vi "Clipper.vi"(8 "error in (no error)":errorcluster) -> (0 "error out":errorcluster)   [LabVIEW 2018, in "MainVIs.lvlib"]
doc: "This template is for the Queued Message Handler design pattern.\n\nThe Event Handling Loop generates messages based on user interface actions.\n\nThe Message Handling Loop processes messages generated by the Event Handling Loop, or by other messages. The messages are string values, so new messages can be added easily to the Message Cases case structure in the Message Handling Loop. Each message cluster can also provide an optional value for Message Data, which is a variant that can be converted to whatever message-specific data is required."
uses:
  MainVIs.lvlib
  <vilib>/Utility/miscctls.llb/LVCursorListTypeDef.ctl
  Analysis Support/Controls/UI Data-Clipper.ctl
  Collection Support/Message Queue/Enqueue Message (Single).vi
  Collection Support/Message Queue/Enqueue Message (Array).vi
  <vilib>/Utility/error.llb/Error Cluster From Error Code.vi
  <vilib>/ErrorRing/Error Ring.xnode
  Collection Support/Message Queue/Message Queue.lvlib
  Collection Support/User Event - Stop/User Event - Stop.lvlib
  CollectionSupport.lvlib
  AnalysisSupport.lvlib
panel:
  in  "Stop Everything?":bool
  out "Right":dbl
  out "Left":dbl
  out "Flow":dynamicdata(graph)
  out "Pressure":dynamicdata(graph)
  out "Audio":dynamicdata(graph)
  out "File Name Display":string
  in  "Remove":bool
  in  "Set Cursors":bool
  in  "Edit File":bool
  out "Message":string
  in  "Save":bool
  in  "Open":bool
  in  "Exit":bool
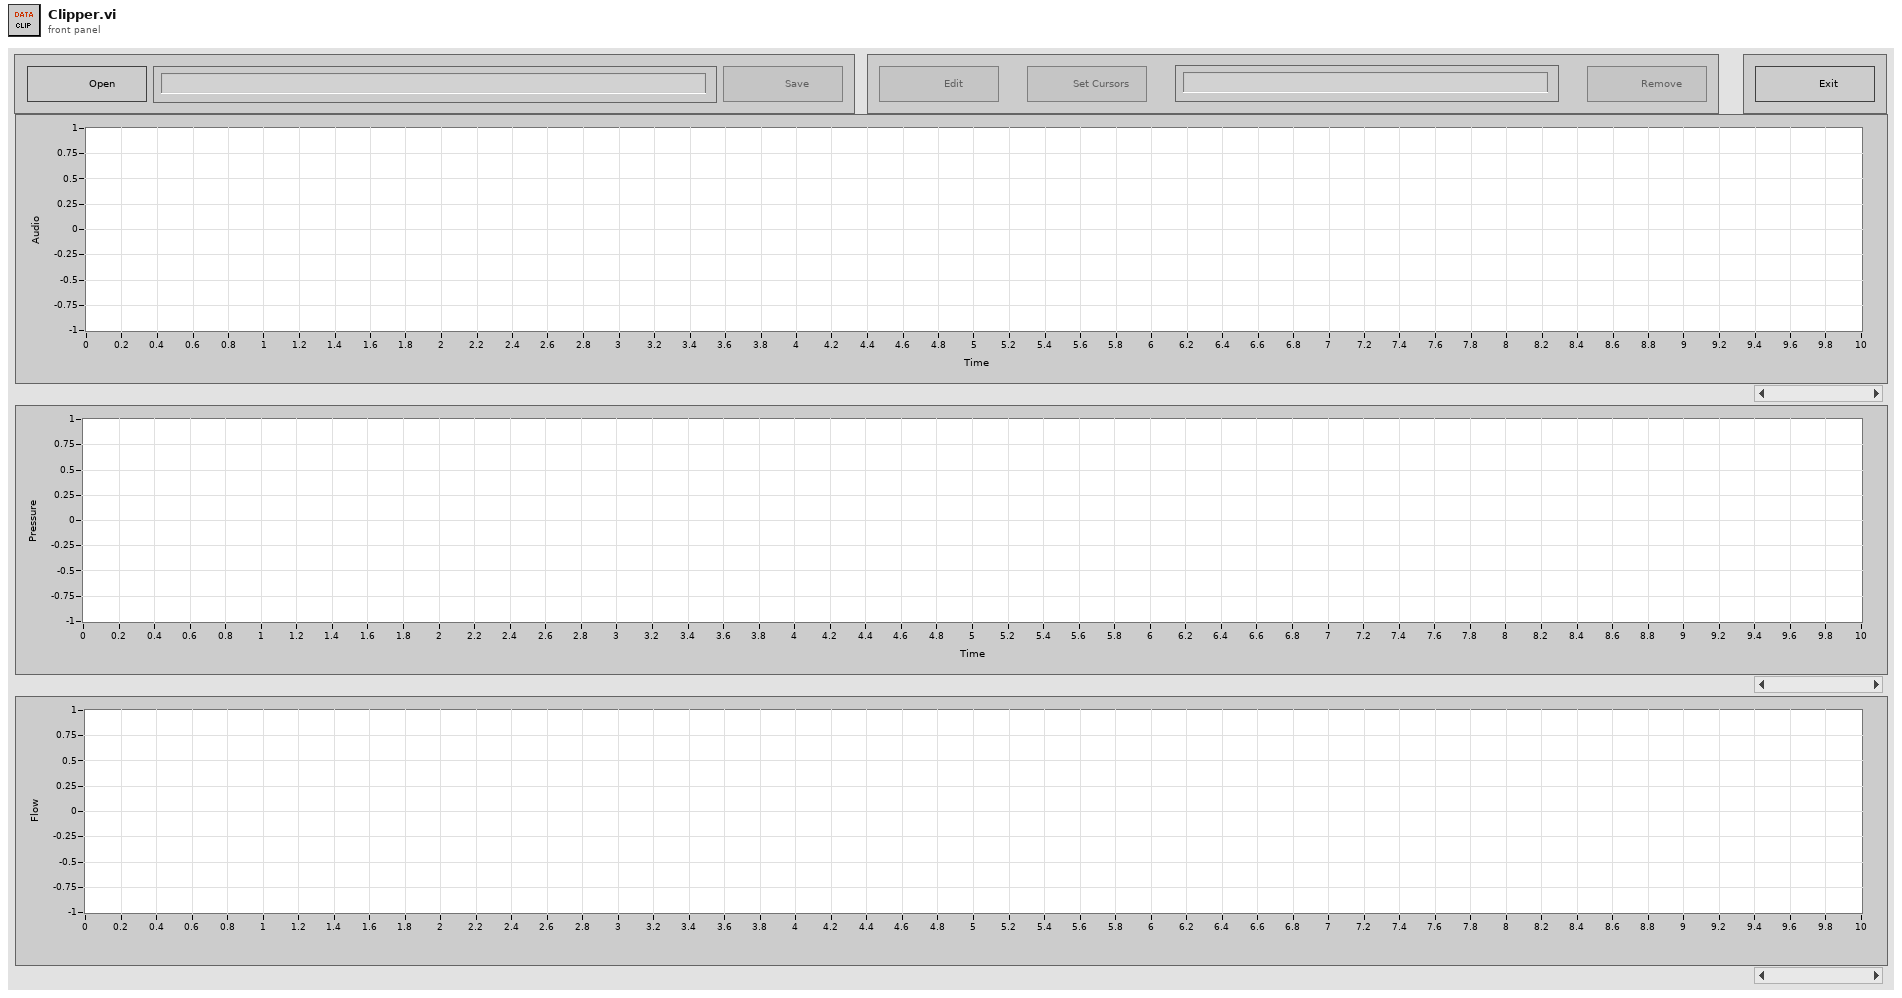
[diagram p1: front panel]
types:
  T1 = typedef "AnalysisSupport.lvlib/UI Data-Clipper.ctl" = cluster{"File Loaded?":bool, "Message":string, "Open Ref":refnum<vi>, "Save Ref":refnum<vi>, "Message Ref":refnum<vi>, "Exit Button Ref":refnum<vi>, "Remove Ref":refnum<vi>, "Set Cursors Ref":refnum<vi>, "Edit File Ref":refnum<vi>, "Audio Ref":refnum<vi>, "Pressure Ref":refnum<vi>, "Flow Ref":refnum<vi>, "Audio":dynamicdata, "Pressure":dynamicdata, "Flow":dynamicdata, "Left Cursor Position":dbl, "Right Cursor Position":dbl, "Cursors Locked?":bool, "File Name Display":string}
  T2 = typedef "LVCursorListTypeDef.ctl" = cluster{"Name":string, "Color":u32, "Style":u8, "Point Style":u8, "Name Visible":bool, "Allow Drag":bool, "Cursor Mode":u32, "Plot":i32, "Index":i32, "Position":cluster{"X":dbl, "Y":dbl}, "X Scale":u32, "Y Scale":u32, "Watch Plots":i32[], "Watch All Plots":bool, "Plot Area":i32, "Label Offset":cluster{"X":dbl, "Y":dbl}}[]
  T3 = typedef "CollectionSupport.lvlib/Message Queue.lvlib/All Message Queues.ctl" = cluster{"UI":refnum<queue>}
  T4 = cluster{"Cursor Constants[0]":cluster{"Name":string, "Color":u32, "Style":u8, "Point Style":u8, "Name Visible":bool, "Allow Drag":bool, "Cursor Mode":u32, "Plot":i32, "Index":i32, "Position":cluster{"X":dbl, "Y":dbl}, "X Scale":u32, "Y Scale":u32, "Watch Plots":i32[], "Watch All Plots":bool, "Plot Area":i32, "Label Offset":cluster{"X":dbl, "Y":dbl}}, "Cursor Constants[1]":cluster{"Name":string, "Color":u32, "Style":u8, "Point Style":u8, "Name Visible":bool, "Allow Drag":bool, "Cursor Mode":u32, "Plot":i32, "Index":i32, "Position":cluster{"X":dbl, "Y":dbl}, "X Scale":u32, "Y Scale":u32, "Watch Plots":i32[], "Watch All Plots":bool, "Plot Area":i32, "Label Offset":cluster{"X":dbl, "Y":dbl}}, "Cursor Constants[2]":cluster{"Name":string, "Color":u32, "Style":u8, "Point Style":u8, "Name Visible":bool, "Allow Drag":bool, "Cursor Mode":u32, "Plot":i32, "Index":i32, "Position":cluster{"X":dbl, "Y":dbl}, "X Scale":u32, "Y Scale":u32, "Watch Plots":i32[], "Watch All Plots":bool, "Plot Area":i32, "Label Offset":cluster{"X":dbl, "Y":dbl}}, "Cursor Constants[3]":cluster{"Name":string, "Color":u32, "Style":u8, "Point Style":u8, "Name Visible":bool, "Allow Drag":bool, "Cursor Mode":u32, "Plot":i32, "Index":i32, "Position":cluster{"X":dbl, "Y":dbl}, "X Scale":u32, "Y Scale":u32, "Watch Plots":i32[], "Watch All Plots":bool, "Plot Area":i32, "Label Offset":cluster{"X":dbl, "Y":dbl}}, "Cursor Constants[4]":cluster{"Name":string, "Color":u32, "Style":u8, "Point Style":u8, "Name Visible":bool, "Allow Drag":bool, "Cursor Mode":u32, "Plot":i32, "Index":i32, "Position":cluster{"X":dbl, "Y":dbl}, "X Scale":u32, "Y Scale":u32, "Watch Plots":i32[], "Watch All Plots":bool, "Plot Area":i32, "Label Offset":cluster{"X":dbl, "Y":dbl}}, "Cursor Constants[5]":cluster{"Name":string, "Color":u32, "Style":u8, "Point Style":u8, "Name Visible":bool, "Allow Drag":bool, "Cursor Mode":u32, "Plot":i32, "Index":i32, "Position":cluster{"X":dbl, "Y":dbl}, "X Scale":u32, "Y Scale":u32, "Watch Plots":i32[], "Watch All Plots":bool, "Plot Area":i32, "Label Offset":cluster{"X":dbl, "Y":dbl}}, "Cursor Constants[6]":cluster{"Name":string, "Color":u32, "Style":u8, "Point Style":u8, "Name Visible":bool, "Allow Drag":bool, "Cursor Mode":u32, "Plot":i32, "Index":i32, "Position":cluster{"X":dbl, "Y":dbl}, "X Scale":u32, "Y Scale":u32, "Watch Plots":i32[], "Watch All Plots":bool, "Plot Area":i32, "Label Offset":cluster{"X":dbl, "Y":dbl}}, "Cursor Constants[7]":cluster{"Name":string, "Color":u32, "Style":u8, "Point Style":u8, "Name Visible":bool, "Allow Drag":bool, "Cursor Mode":u32, "Plot":i32, "Index":i32, "Position":cluster{"X":dbl, "Y":dbl}, "X Scale":u32, "Y Scale":u32, "Watch Plots":i32[], "Watch All Plots":bool, "Plot Area":i32, "Label Offset":cluster{"X":dbl, "Y":dbl}}, "Cursor Constants[8]":cluster{"Name":string, "Color":u32, "Style":u8, "Point Style":u8, "Name Visible":bool, "Allow Drag":bool, "Cursor Mode":u32, "Plot":i32, "Index":i32, "Position":cluster{"X":dbl, "Y":dbl}, "X Scale":u32, "Y Scale":u32, "Watch Plots":i32[], "Watch All Plots":bool, "Plot Area":i32, "Label Offset":cluster{"X":dbl, "Y":dbl}}}
  T5 = cluster{"Name":string, "Color":u32, "Style":u8, "Point Style":u8, "Name Visible":bool, "Allow Drag":bool, "Cursor Mode":u32, "Plot":i32, "Index":i32, "Position":cluster{"X":dbl, "Y":dbl}, "X Scale":u32, "Y Scale":u32, "Watch Plots":i32[], "Watch All Plots":bool, "Plot Area":i32, "Label Offset":cluster{"X":dbl, "Y":dbl}}[]
  T6 = cluster{"CrsrList[0]":cluster{"Name":string, "Color":u32, "Style":u8, "Point Style":u8, "Name Visible":bool, "Allow Drag":bool, "Cursor Mode":u32, "Plot":i32, "Index":i32, "Position":cluster{"X":dbl, "Y":dbl}, "X Scale":u32, "Y Scale":u32, "Watch Plots":i32[], "Watch All Plots":bool, "Plot Area":i32, "Label Offset":cluster{"X":dbl, "Y":dbl}}, "CrsrList[1]":cluster{"Name":string, "Color":u32, "Style":u8, "Point Style":u8, "Name Visible":bool, "Allow Drag":bool, "Cursor Mode":u32, "Plot":i32, "Index":i32, "Position":cluster{"X":dbl, "Y":dbl}, "X Scale":u32, "Y Scale":u32, "Watch Plots":i32[], "Watch All Plots":bool, "Plot Area":i32, "Label Offset":cluster{"X":dbl, "Y":dbl}}, "CrsrList[2]":cluster{"Name":string, "Color":u32, "Style":u8, "Point Style":u8, "Name Visible":bool, "Allow Drag":bool, "Cursor Mode":u32, "Plot":i32, "Index":i32, "Position":cluster{"X":dbl, "Y":dbl}, "X Scale":u32, "Y Scale":u32, "Watch Plots":i32[], "Watch All Plots":bool, "Plot Area":i32, "Label Offset":cluster{"X":dbl, "Y":dbl}}, "CrsrList[3]":cluster{"Name":string, "Color":u32, "Style":u8, "Point Style":u8, "Name Visible":bool, "Allow Drag":bool, "Cursor Mode":u32, "Plot":i32, "Index":i32, "Position":cluster{"X":dbl, "Y":dbl}, "X Scale":u32, "Y Scale":u32, "Watch Plots":i32[], "Watch All Plots":bool, "Plot Area":i32, "Label Offset":cluster{"X":dbl, "Y":dbl}}, "CrsrList[4]":cluster{"Name":string, "Color":u32, "Style":u8, "Point Style":u8, "Name Visible":bool, "Allow Drag":bool, "Cursor Mode":u32, "Plot":i32, "Index":i32, "Position":cluster{"X":dbl, "Y":dbl}, "X Scale":u32, "Y Scale":u32, "Watch Plots":i32[], "Watch All Plots":bool, "Plot Area":i32, "Label Offset":cluster{"X":dbl, "Y":dbl}}, "CrsrList[5]":cluster{"Name":string, "Color":u32, "Style":u8, "Point Style":u8, "Name Visible":bool, "Allow Drag":bool, "Cursor Mode":u32, "Plot":i32, "Index":i32, "Position":cluster{"X":dbl, "Y":dbl}, "X Scale":u32, "Y Scale":u32, "Watch Plots":i32[], "Watch All Plots":bool, "Plot Area":i32, "Label Offset":cluster{"X":dbl, "Y":dbl}}, "CrsrList[6]":cluster{"Name":string, "Color":u32, "Style":u8, "Point Style":u8, "Name Visible":bool, "Allow Drag":bool, "Cursor Mode":u32, "Plot":i32, "Index":i32, "Position":cluster{"X":dbl, "Y":dbl}, "X Scale":u32, "Y Scale":u32, "Watch Plots":i32[], "Watch All Plots":bool, "Plot Area":i32, "Label Offset":cluster{"X":dbl, "Y":dbl}}, "CrsrList[7]":cluster{"Name":string, "Color":u32, "Style":u8, "Point Style":u8, "Name Visible":bool, "Allow Drag":bool, "Cursor Mode":u32, "Plot":i32, "Index":i32, "Position":cluster{"X":dbl, "Y":dbl}, "X Scale":u32, "Y Scale":u32, "Watch Plots":i32[], "Watch All Plots":bool, "Plot Area":i32, "Label Offset":cluster{"X":dbl, "Y":dbl}}, "CrsrList[8]":cluster{"Name":string, "Color":u32, "Style":u8, "Point Style":u8, "Name Visible":bool, "Allow Drag":bool, "Cursor Mode":u32, "Plot":i32, "Index":i32, "Position":cluster{"X":dbl, "Y":dbl}, "X Scale":u32, "Y Scale":u32, "Watch Plots":i32[], "Watch All Plots":bool, "Plot Area":i32, "Label Offset":cluster{"X":dbl, "Y":dbl}}}
  T7 = typedef "eventvkey.ctl" = enum16{"ASCII", "Enter", "Return", "Shift", "Ctrl", "Alt", "Cmd", "Opt", "Caps", "NumLock", "Clear", "Break", "Up", "Down", "Left", "Right", "Insert", "Delete", "Home", "End", "PageUp", "PageDown", "Escape", "Help", "Pause", "ScrollLock", "F1", "F2", "F3", "F4", "F5", "F6", "F7", "F8", "F9", "F10", "F11", "F12", "F13", "F14", "F15", "F16", "F17", "F18", "F19", "F20", "F21", "F22", "F23", "F24", "Play", "VolumeUp", "VolumeDown", "Mute", "Two Byte Char"}
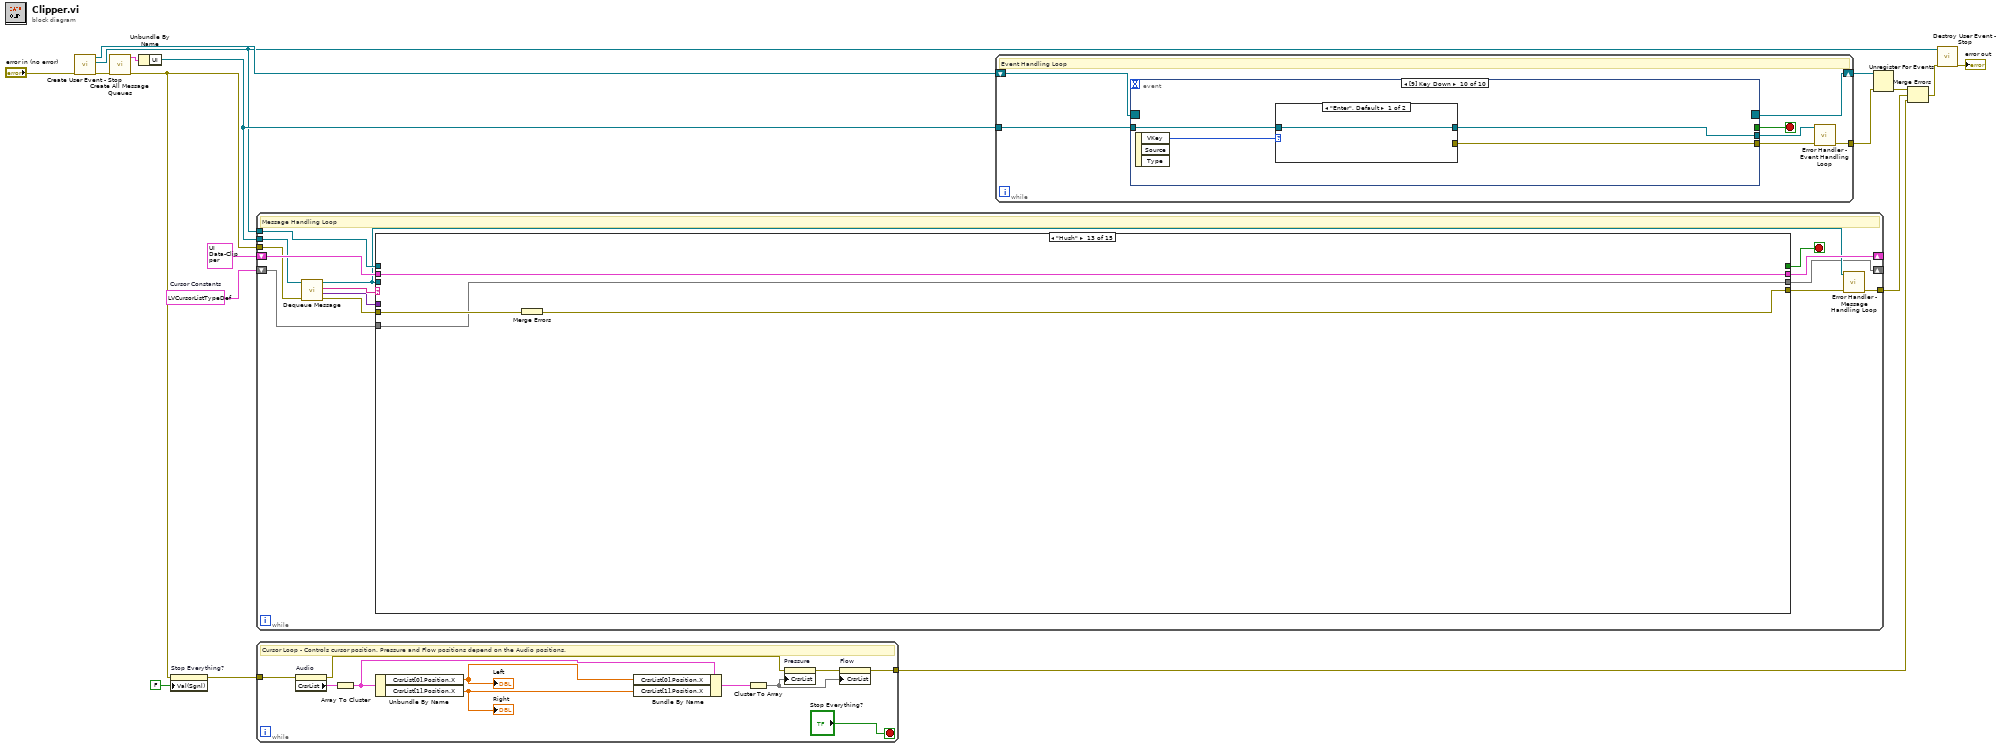
[diagram p0: block diagram]
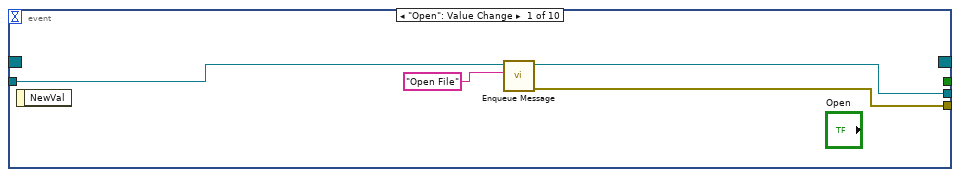
[diagram p2: hidden frame]
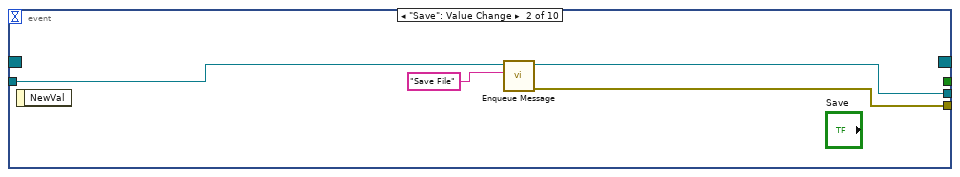
[diagram p3: hidden frame]
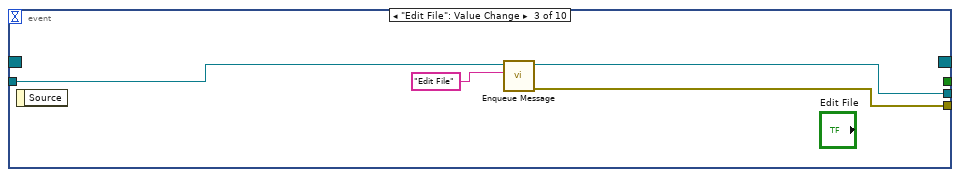
[diagram p4: hidden frame]
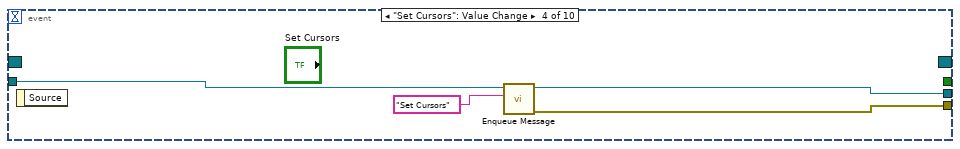
[diagram p5: hidden frame]
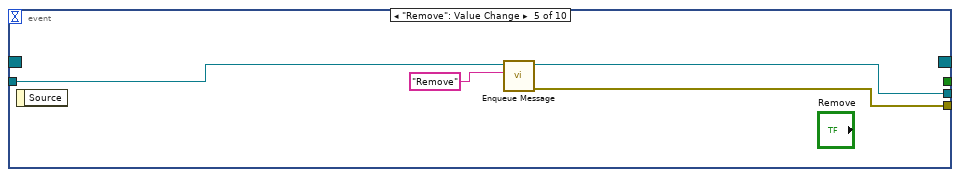
[diagram p6: hidden frame]
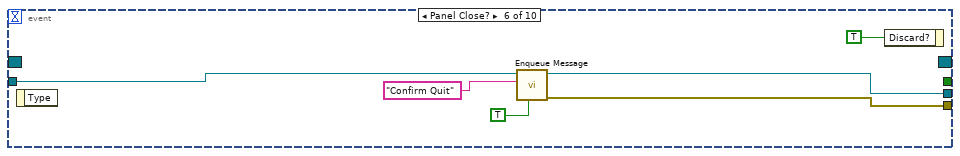
[diagram p7: hidden frame]
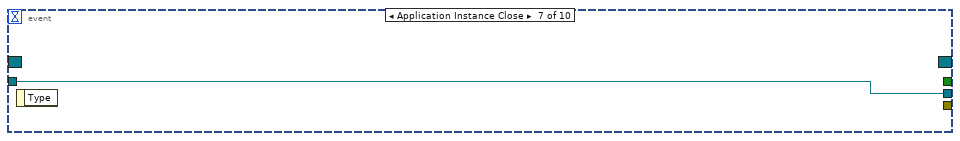
[diagram p8: hidden frame]
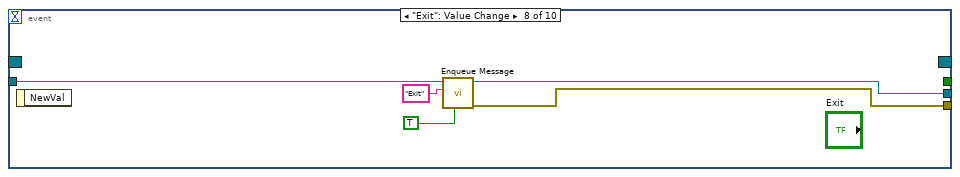
[diagram p9: hidden frame]
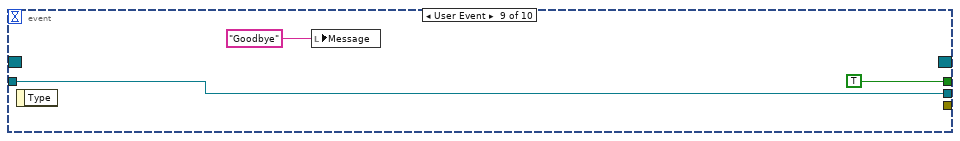
[diagram p10: hidden frame]
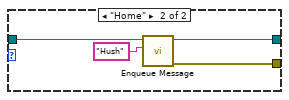
[diagram p11: hidden frame]
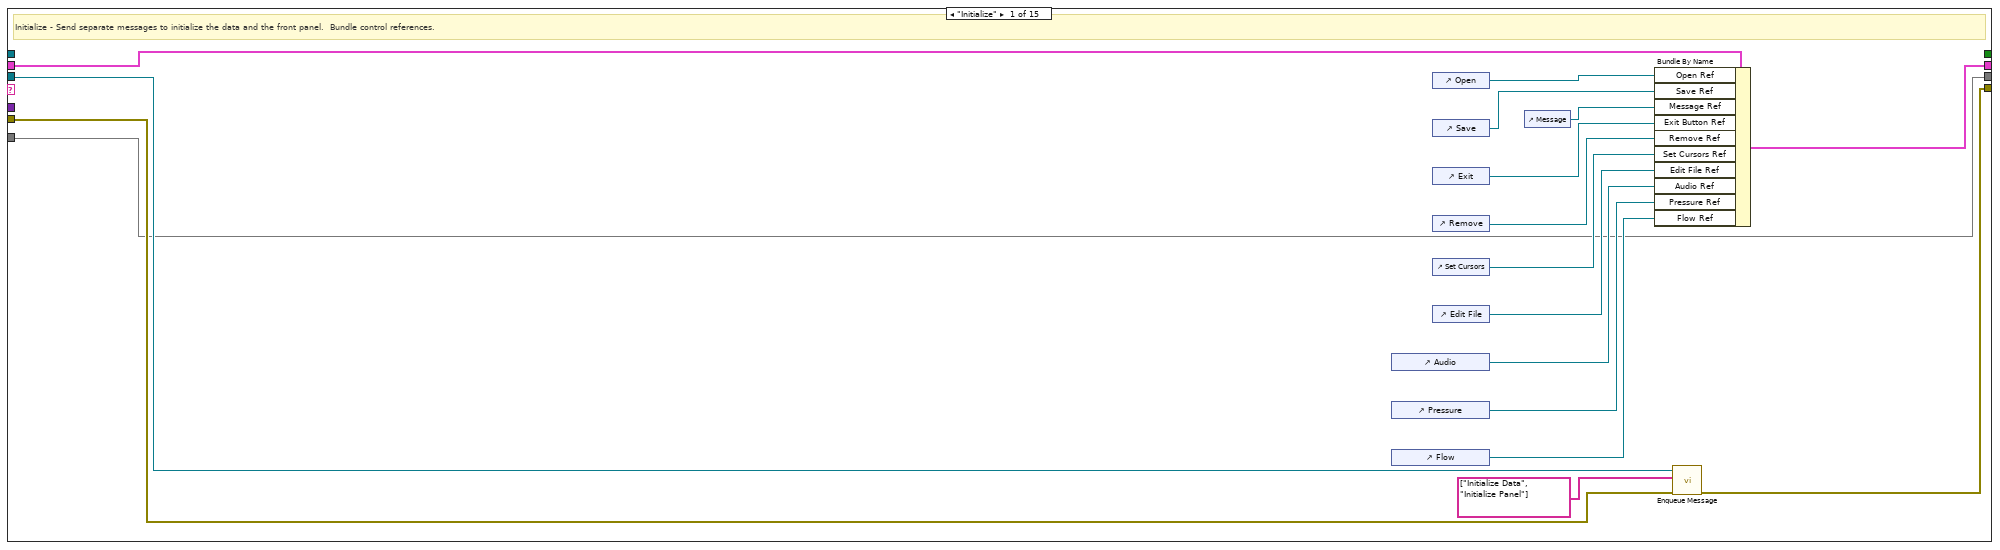
[diagram p12: hidden frame]
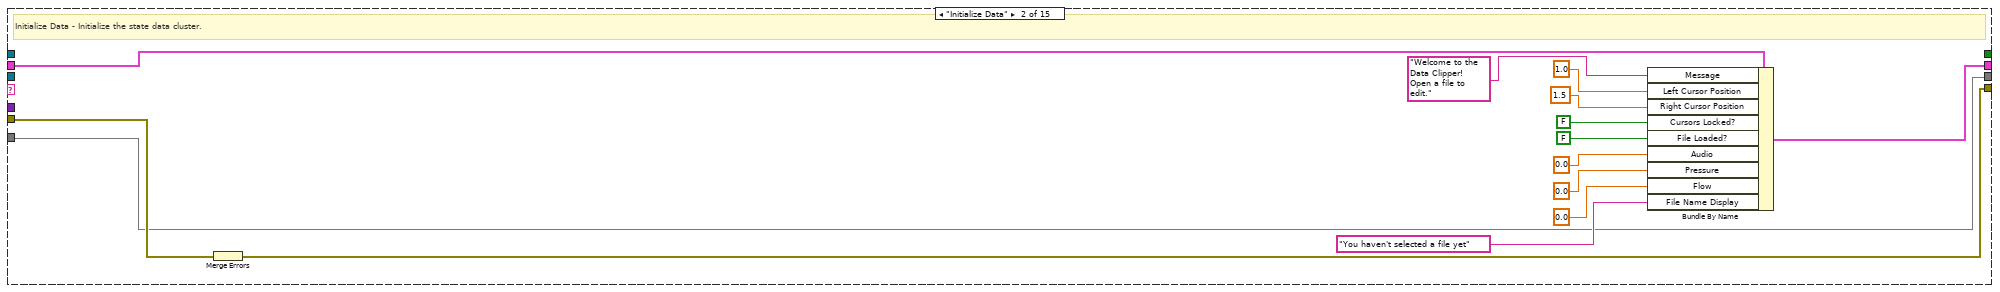
[diagram p13: hidden frame]
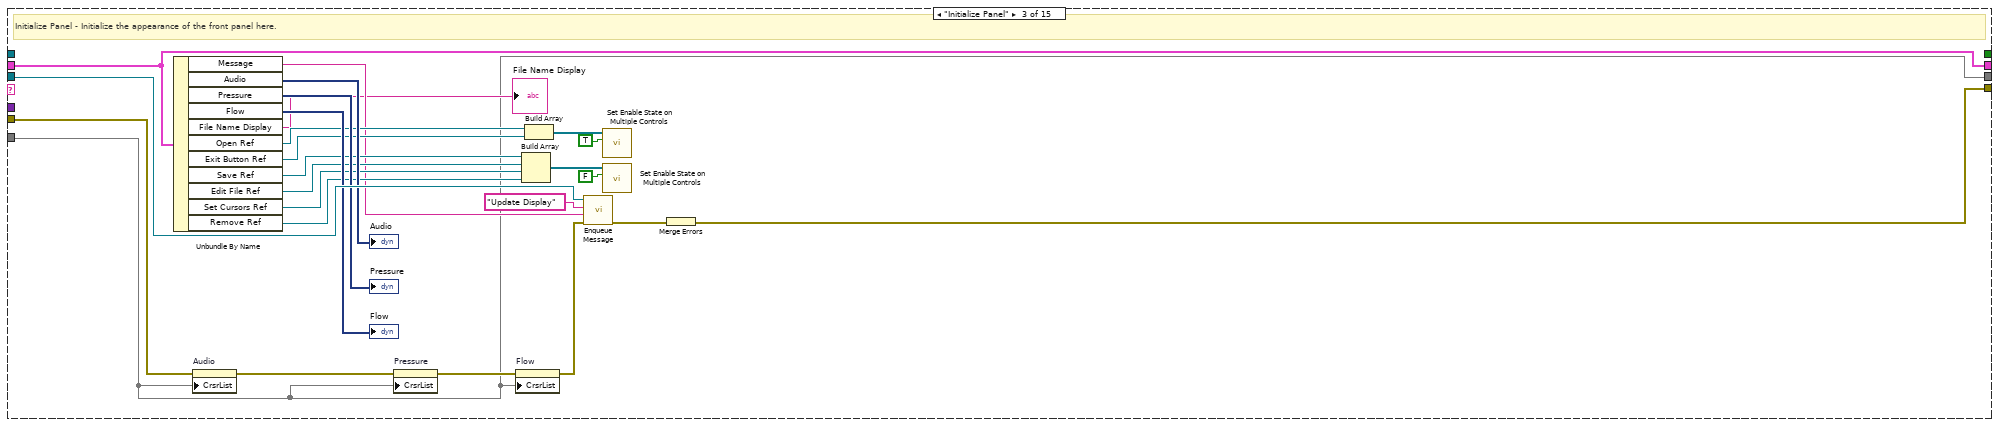
[diagram p14: hidden frame]
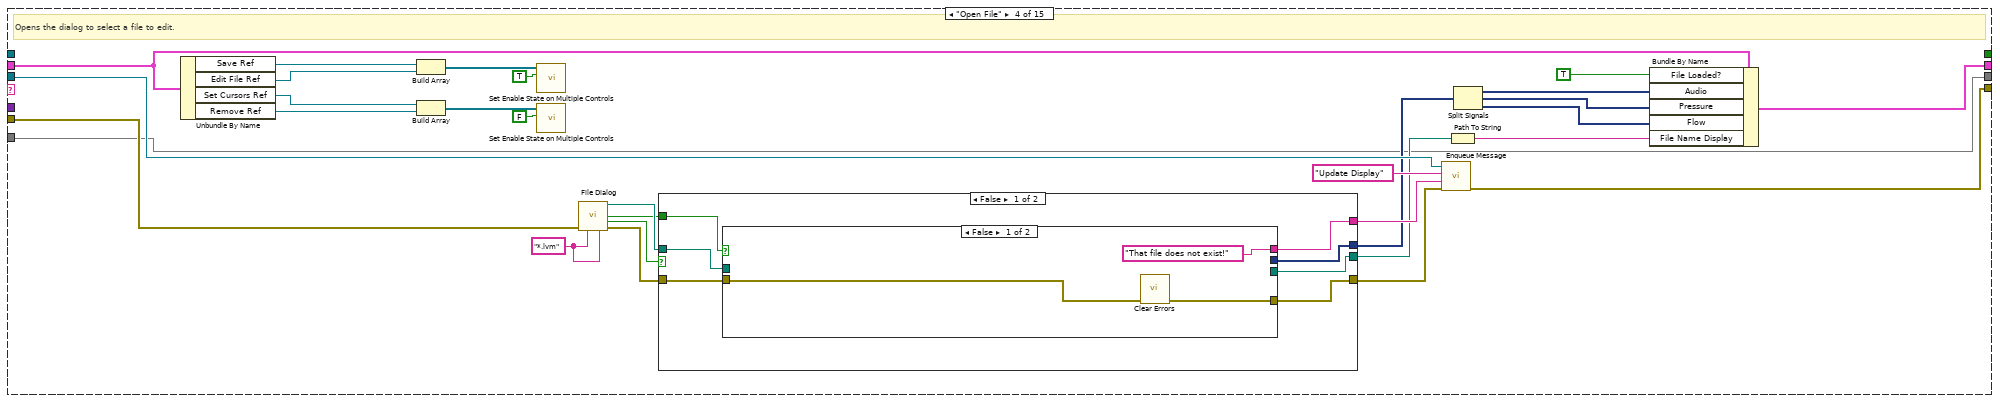
[diagram p15: hidden frame]
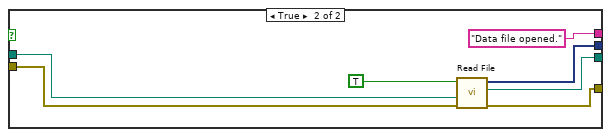
[diagram p16: hidden frame]
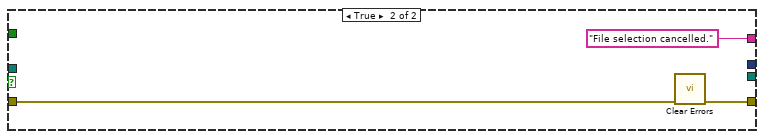
[diagram p17: hidden frame]
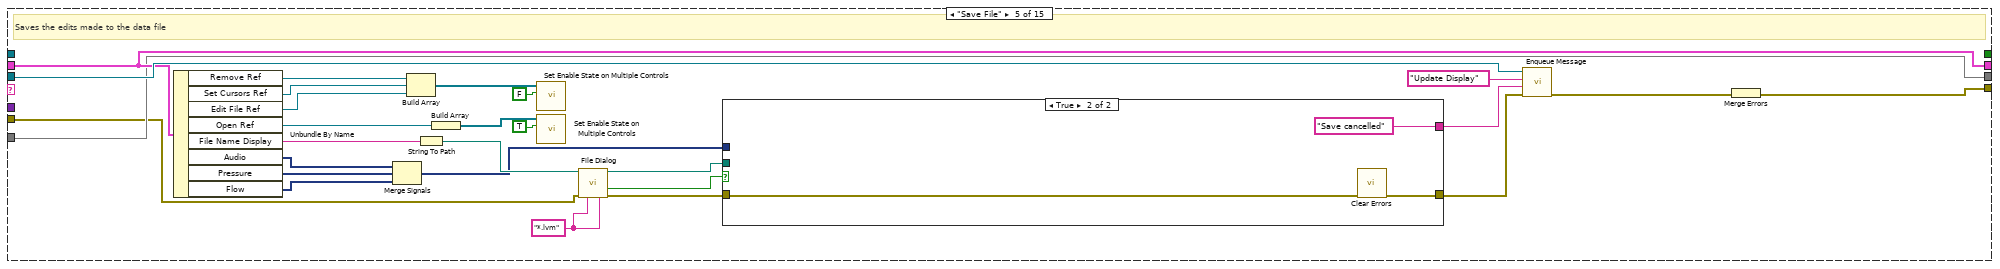
[diagram p18: hidden frame]
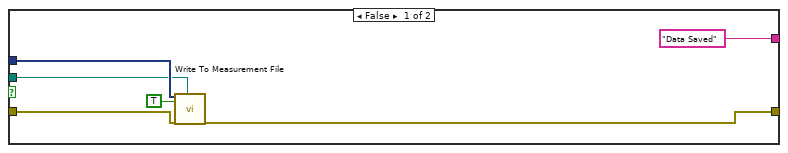
[diagram p19: hidden frame]
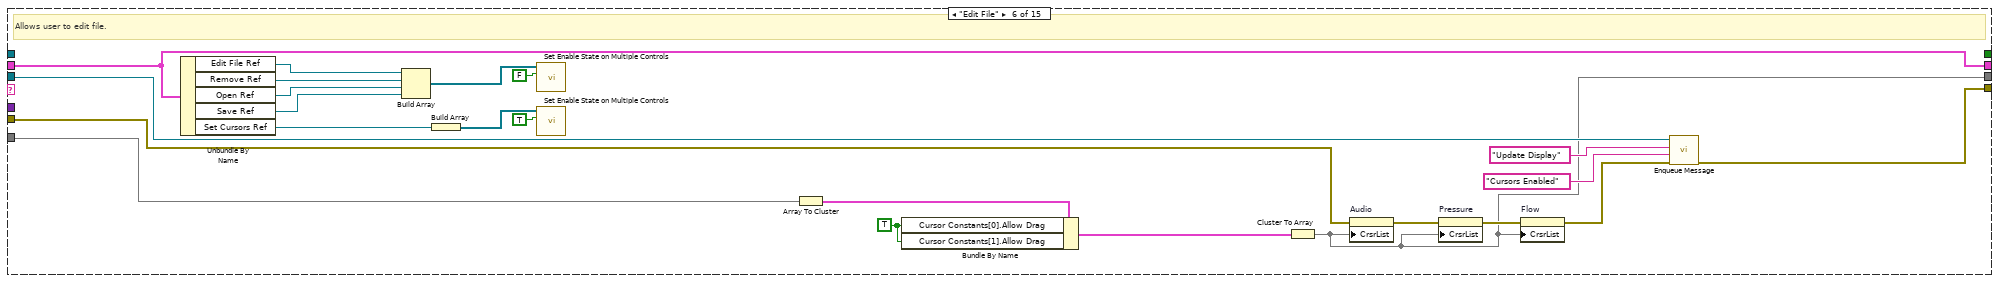
[diagram p20: hidden frame]
diagram:
  w9 = T2 [{"Name"="Left", "Color"=255, "Style"=2, "Point Style"=1, "Name Visible"=FALSE, "Allow Drag"=FALSE, "Cursor Mode"=0, "Plot"=0, "Index"=0, "Position"={"X"=2.0, "Y"=0.0}, "X Scale"=0, "Y Scale"=0, "Watch Plots"=[], "Watch All Plots"=FALSE, "Plot Area"=0, "Label Offset"={"X"=0.0, "Y"=0.0}}, {"Name"="Right", "Color"=13107455, "Style"=2, "Point Style"=1, "Name Visible"=FALSE, "Allow Drag"=FALSE, "Cursor Mode"=0, "Plot"=0, "Index"=0, "Position"={"X"=3.0, "Y"=0.0}, "X Scale"=0, "Y Scale"=0, "Watch Plots"=[], "Watch All Plots"=FALSE, "Plot Area"=0, "Label Offset"={"X"=0.0, "Y"=0.0}}]  # Cursor Constants
  n1 = call "Create User Event - Stop.vi"("error in (no error)"="error in (no error)") -> ("error out"=w8:errorcluster, "User Event - Stop"=w14:refnum<user-event>, "Stop Event Registration Refnum"=w15:refnum<event-registration>)  [unwired: 8 in]
  n2 = call "Create All Message Queues.vi"("error in (no error)"=w8) -> ("error out"=w5:errorcluster, "Message Queues out"=w18:T3)  [unwired: 9 in]
  n3 = Unbundle By Name(w18) -> ("UI"=w16:refnum<queue>)
  n4 = property on="Stop Everything?" class="Bool (strict)"(error in=w5, "Val(Sgnl)"=FALSE ("Value (Signaling)")) -> (error out=w6:errorcluster)  [unwired: 1 in, 1 out]
  n5 = while {
    tunnel: w16 -> [w24]
    shift-right: [w31] -> _
    shift-left: T1 {"File Loaded?"=FALSE, "Message"="", "Open Ref"=refnum, "Save Ref"=refnum, "Message Ref"=refnum, "Exit Button Ref"=refnum, "Remove Ref"=refnum, "Set Cursors Ref"=refnum, "Edit File Ref"=refnum, "Audio Ref"=refnum, "Pressure Ref"=refnum, "Flow Ref"=refnum, "Audio"=[], "Pressure"=[], "Flow"=[], "Left Cursor Position"=0.0, "Right Cursor Position"=0.0, "Cursors Locked?"=FALSE, "File Name Display"=""} ("UI Data") -> [w32]
    tunnel: w14 -> [w29]
    tunnel: w5 -> [w28]
    tunnel: [w22] -> w17
    shift-right: [w19] -> _
    shift-left: w9 -> [w20]
    stop <- w30 stop-if-true
    # "Message Handling Loop"
    n6 = call "Dequeue Message.vi"("error in (no error)"=w28, "Message Queue"=w24) -> ("error out"=w27:errorcluster, "Message Data"=w25:variant, "Message"=w26:string, "dup Message Queue"=w23:refnum<queue>)  [unwired: 6 in]
    n7 = case "Message Cases" shown="\"Hush\"" w26 {
      selector: w26 -> [_ _ _ _ _ _ _ _ _ _ _ _ _ _ w293]
      tunnel: w23 -> [w47 _ w86 w117 w162 w194 w214 w238 _ w257 w269 _ _ w291 _]
      tunnel: w27 -> [w48 w63 w66 w98 w149 w176 w200 w227 w252 w265 w273 w277 w281 w286 _]
      tunnel: [w49 w51 w87 w89 w164 w193 w213 w239 w253 w258 w271 w275 w279 w287 w294] -> w21
      tunnel: w32 -> [w46 w62 w88 w114 w160 w184 w210 w231 w247 w264 w272 w276 w280 w290 w295]
      tunnel: [w45 w61 w88 w112 w160 w184 w210 w230 w247 w264 w272 w276 w280 w290 w295] -> w31
      tunnel: [_ _ _ _ _ _ _ _ _ _ _ _ _ TRUE _] -> w30
      tunnel: w25 -> [_ _ _ _ _ _ _ _ w251 w263 _ _ _ _ _]
      tunnel: w29 -> [_ _ _ _ _ _ _ _ _ _ _ _ _ w285 _]
      tunnel: w20 -> [w33 w50 w64 w94 w151 w182 w204 w233 w242 w254 w266 w274 w278 w282 w292]
      tunnel: [w33 w50 w64 w94 w151 w175 w199 w233 w242 w254 w266 w274 w278 w282 w292] -> w19
      frame "Initialize" {
        # "Initialize - Send separate messages to initialize the data and the front panel.  Bundle control references."
        n8 = control-ref of="Audio"() -> (w37:refnum<vi>)
        n9 = control-ref of="Pressure"() -> (w36:refnum<vi>)
        n10 = control-ref of="Flow"() -> (w34:refnum<vi>)
        n11 = control-ref of="Open"() -> (w35:refnum<vi>)
        n12 = control-ref of="Save"() -> (w43:refnum<vi>)
        n13 = control-ref of="Exit"() -> (w41:refnum<vi>)
        n14 = control-ref of="Remove"() -> (w40:refnum<vi>)
        n15 = control-ref of="Set Cursors"() -> (w39:refnum<vi>)
        n16 = control-ref of="Edit File"() -> (w38:refnum<vi>)
        n17 = control-ref of="Message"() -> (w42:refnum<vi>)
        n18 = Bundle By Name(cluster=w46, "Open Ref"=w35, "Save Ref"=w43, "Message Ref"=w42, "Exit Button Ref"=w41, "Remove Ref"=w40, "Set Cursors Ref"=w39, "Edit File Ref"=w38, "Audio Ref"=w37, "Pressure Ref"=w36, "Flow Ref"=w34) -> (w45:T1)
        n19 = call-poly "Enqueue Message.vi"("error in (no error)"=w48, "Message Array"=string[] ["Initialize Data", "Initialize Panel"], "Message Queue"=w47) -> ("error out"=w49:errorcluster)  [unwired: 7 in, 1 out]
      }
      frame "Initialize Data" {
        # "Initialize Data - Initialize the state data cluster."
        n20 = Merge Errors(w63) -> (w51:errorcluster)
        n21 = Bundle By Name(cluster=w62, "Message"="Welcome to the Data Clipper! Open a file to edit." ("Initial Message"), "Left Cursor Position"=1.0, "Right Cursor Position"=1.5, "Cursors Locked?"=FALSE, "File Loaded?"=FALSE, "Audio"=0.0, "Pressure"=0.0, "Flow"=0.0, "File Name Display"="You haven't selected a file yet") -> (w61:T1)
      }
      frame "Initialize Panel" {
        # "Initialize Panel - Initialize the appearance of the front panel here."
        n22 = Unbundle By Name(w88) -> ("Message"=w70:string, "Audio"=→"Audio":dynamicdata, "Pressure"=→"Pressure":dynamicdata, "Flow"=→"Flow":dynamicdata, "File Name Display"=→"File Name Display":string, "Open Ref"=w78:refnum<vi>, "Exit Button Ref"=w77:refnum<vi>, "Save Ref"=w76:refnum<vi>, "Edit File Ref"=w75:refnum<vi>, "Set Cursors Ref"=w74:refnum<vi>, "Remove Ref"=w73:refnum<vi>)
        n23 = property on="Audio" class="WFGraph (strict)"(error in=w66, "CrsrList"=w64) -> (error out=w68:errorcluster)  [unwired: 1 in, 1 out]
        n24 = property on="Pressure" class="WFGraph (strict)"(error in=w68, "CrsrList"=w64) -> (error out=w67:errorcluster)  [unwired: 1 in, 1 out]
        n25 = property on="Flow" class="WFGraph (strict)"(error in=w67, "CrsrList"=w64) -> (error out=w65:errorcluster)  [unwired: 1 in, 1 out]
        n26 = Build Array(w76, w75, w74, w73) -> (w72:refnum<vi>[])
        n27 = Build Array(w78, w77) -> (w79:refnum<vi>[])
        n28 = call-poly "Enqueue Message.vi"("error in (no error)"=w65, "Message Data"=w70, "Message"="Update Display", "Message Queue"=w86) -> ("error out"=w85:errorcluster)  [unwired: 6 in, 1 out]
        n29 = call "Set Enable State on Multiple Controls.vi"("Enable?"=TRUE, "Controls"=w79) -> ()  [unwired: 10 in]
        n30 = call "Set Enable State on Multiple Controls.vi"("Enable?"=FALSE, "Controls"=w72) -> ()  [unwired: 10 in]
        n31 = Merge Errors(w85) -> (w87:errorcluster)
      }
      frame "Open File" {
        w107 = "*.lvm" ("pattern label")
        # "Opens the dialog to select a file to edit."
        n32 = Unbundle By Name(w114) -> ("Save Ref"=w109:refnum<vi>, "Edit File Ref"=w110:refnum<vi>, "Set Cursors Ref"=w93:refnum<vi>, "Remove Ref"=w90:refnum<vi>)
        n33 = Build Array(w109, w110) -> (w108:refnum<vi>[])
        n34 = Build Array(w93, w90) -> (w92:refnum<vi>[])
        n35 = call "Set Enable State on Multiple Controls.vi"("Enable?"=TRUE, "Controls"=w108) -> ()  [unwired: 10 in]
        n36 = call "Set Enable State on Multiple Controls.vi"("Enable?"=FALSE, "Controls"=w92) -> ()  [unwired: 10 in]
        n37 = call "File Dialog"("error in"=w98, "pattern (all files)"=w107, "pattern label"=w107) -> ("selected path"=w105:path, "exists"=w95:bool, "cancelled"=w96:bool, "error out"=w106:errorcluster)  [unwired: 9 in]
        n38 = case shown="False" w96 {
          tunnel: [w124 "File selection cancelled." ("\"Do Something\" button pressed")] -> w115
          tunnel: w106 -> [w123 w136]
          tunnel: w105 -> [w122 _]
          tunnel: [w121 _] -> w104
          tunnel: [w120 _] -> w103
          tunnel: [w119 w135] -> w97
          tunnel: w95 -> [w118 _]
          frame False {
            n39 = case shown="False" w118 {
              tunnel: ["That file does not exist!" ("\"Do Something\" button pressed") "Data file opened." ("\"Do Something\" button pressed")] -> w124
              tunnel: w123 -> [w126 w132]
              tunnel: w122 -> [_ w131]
              tunnel: [_ w130] -> w121
              tunnel: [_ w129] -> w120
              tunnel: [w125 w128] -> w119
              frame False {
                n40 = call <vilib>:"Clear Errors.vi"("error in (no error)"=w126) -> ("error out"=w125:errorcluster)  [unwired: 5 in, 1 out]
              }
              frame True {
                n41 = call "Read File"("error in (no error)"=w132, "Filename"=w131, "Reset"=TRUE) -> ("error out"=w128:errorcluster, "Filename Out"=w130:path, "Signals"=w129:dynamicdata)  [unwired: 3 in, 3 out]
              }
            }
          }
          frame True {
            n42 = call <vilib>:"Clear Errors.vi"("error in (no error)"=w136) -> ("error out"=w135:errorcluster)  [unwired: 5 in, 1 out]
          }
        }
        n43 = call-poly "Enqueue Message.vi"("error in (no error)"=w97, "Message Data"=w115, "Message"="Update Display", "Message Queue"=w117) -> ("error out"=w89:errorcluster)  [unwired: 6 in, 1 out]
        n44 = Path To String(path=w104) -> (string=w99:string)
        n45 = Split Signals(w103) -> (w102:dynamicdata, w101:dynamicdata, w100:dynamicdata)  [unwired: 3 in]
        n46 = Bundle By Name(cluster=w114, "File Loaded?"=TRUE, "Audio"=w102, "Pressure"=w101, "Flow"=w100, "File Name Display"=w99) -> (w112:T1)
      }
      frame "Save File" {
        w147 = "*.lvm" ("pattern (all files)")
        # "Saves the edits made to the data file"
        n47 = Unbundle By Name(w160) -> ("Remove Ref"=w157:refnum<vi>, "Set Cursors Ref"=w156:refnum<vi>, "Edit File Ref"=w155:refnum<vi>, "Open Ref"=w152:refnum<vi>, "File Name Display"=w150:string, "Audio"=w144:dynamicdata, "Pressure"=w143:dynamicdata, "Flow"=w142:dynamicdata)
        n48 = Merge Signals(w144, w143, w142) -> (w141:dynamicdata)
        n49 = Build Array(w157, w156, w155) -> (w159:refnum<vi>[])
        n50 = String To Path(string=w150) -> (path=w148:path)
        n51 = Build Array(w152) -> (w154:refnum<vi>[])
        n52 = call "Set Enable State on Multiple Controls.vi"("Enable?"=FALSE, "Controls"=w159) -> ()  [unwired: 10 in]
        n53 = call "Set Enable State on Multiple Controls.vi"("Enable?"=TRUE, "Controls"=w154) -> ()  [unwired: 10 in]
        n54 = call "File Dialog"("start path"=w148, "error in"=w149, "pattern (all files)"=w147, "pattern label"=w147) -> ("selected path"=w140:path, "cancelled"=w139:bool, "error out"=w146:errorcluster)  [unwired: 8 in, 1 out]
        n55 = case shown="True" w139 {
          tunnel: w146 -> [w170 w172]
          tunnel: [w169 w171] -> w145
          tunnel: w141 -> [w168 _]
          tunnel: w140 -> [w166 _]
          tunnel: ["Data Saved" ("\"Do Something Else\" button pressed") "Save cancelled" ("\"Do Something Else\" button pressed")] -> w138
          frame False {
            n56 = call "Write To Measurement File"("Signals"=w168, "Reset"=TRUE, "error in (no error)"=w170, "Filename"=w166) -> ("error out"=w169:errorcluster)  [unwired: 13 in, 2 out]
          }
          frame True {
            n57 = call <vilib>:"Clear Errors.vi"("error in (no error)"=w172) -> ("error out"=w171:errorcluster)  [unwired: 5 in, 1 out]
          }
        }
        n58 = call-poly "Enqueue Message.vi"("error in (no error)"=w145, "Message Data"=w138, "Message"="Update Display", "Message Queue"=w162) -> ("error out"=w163:errorcluster)  [unwired: 6 in, 1 out]
        n59 = Merge Errors(w163) -> (w164:errorcluster)
      }
      frame "Edit File" {
        w183 = TRUE ("CrsrList[0].Allow Drag")
        # "Allows user to edit file."
        n60 = Unbundle By Name(w184) -> ("Edit File Ref"=w174:refnum<vi>, "Remove Ref"=w185:refnum<vi>, "Open Ref"=w190:refnum<vi>, "Save Ref"=w189:refnum<vi>, "Set Cursors Ref"=w186:refnum<vi>)
        n61 = Build Array(w174, w185, w190, w189) -> (w192:refnum<vi>[])
        n62 = Build Array(w186) -> (w188:refnum<vi>[])
        n63 = call "Set Enable State on Multiple Controls.vi"("Enable?"=FALSE, "Controls"=w192) -> ()  [unwired: 10 in]
        n64 = call "Set Enable State on Multiple Controls.vi"("Enable?"=TRUE, "Controls"=w188) -> ()  [unwired: 10 in]
        n65 = Array To Cluster(array=w182) -> (cluster=w181:T4)
        n66 = Bundle By Name(cluster=w181, "Cursor Constants[0].Allow Drag"=w183, "Cursor Constants[1].Allow Drag"=w183) -> (w180:T4)
        n67 = Cluster To Array(cluster=w180) -> (array=w175:T5)
        n68 = property on="Audio" class="WFGraph (strict)"(error in=w176, "CrsrList"=w175) -> (error out=w179:errorcluster)  [unwired: 1 in, 1 out]
        n69 = property on="Pressure" class="WFGraph (strict)"(error in=w179, "CrsrList"=w175) -> (error out=w178:errorcluster)  [unwired: 1 in, 1 out]
        n70 = property on="Flow" class="WFGraph (strict)"(error in=w178, "CrsrList"=w175) -> (error out=w177:errorcluster)  [unwired: 1 in, 1 out]
        n71 = call-poly "Enqueue Message.vi"("error in (no error)"=w177, "Message Data"="Cursors Enabled" ("\"Do Something Else\" button pressed"), "Message"="Update Display", "Message Queue"=w194) -> ("error out"=w193:errorcluster)  [unwired: 6 in, 1 out]
      }
      frame "Set Cursors" {
        w207 = FALSE ("CrsrList[0].Allow Drag")
        (unwired) FALSE ("element")
        # "Locks the cursors."
        n72 = Unbundle By Name(w210) -> ("Edit File Ref"=w209:refnum<vi>, "Remove Ref"=w208:refnum<vi>)
        n73 = Build Array(w209, w208) -> (w212:refnum<vi>[])
        n74 = call "Set Enable State on Multiple Controls.vi"("Enable?"=TRUE, "Controls"=w212) -> ()  [unwired: 10 in]
        n75 = Array To Cluster(array=w204) -> (cluster=w205:T4)
        n76 = local read "Right"() -> (w197:dbl)
        n77 = local read "Left"() -> (w198:dbl)
        n78 = Bundle By Name(cluster=w205, "Cursor Constants[0].Allow Drag"=w207, "Cursor Constants[1].Allow Drag"=w207, "Cursor Constants[0].Position.X"=w198, "Cursor Constants[1].Position.X"=w197) -> (w206:T4)
        n79 = Cluster To Array(cluster=w206) -> (array=w199:T5)
        n80 = property on="Audio" class="WFGraph (strict)"(error in=w200, "CrsrList"=w199) -> (error out=w203:errorcluster)  [unwired: 1 in, 1 out]
        n81 = property on="Pressure" class="WFGraph (strict)"(error in=w203, "CrsrList"=w199) -> (error out=w202:errorcluster)  [unwired: 1 in, 1 out]
        n82 = property on="Flow" class="WFGraph (strict)"(error in=w202, "CrsrList"=w199) -> (error out=w201:errorcluster)  [unwired: 1 in, 1 out]
        n83 = call-poly "Enqueue Message.vi"("error in (no error)"=w201, "Message Data"="Cursors Locked" ("\"Do Something Else\" button pressed"), "Message"="Update Display", "Message Queue"=w214) -> ("error out"=w213:errorcluster)  [unwired: 6 in, 1 out]
      }
      frame "Remove" {
        # "Opens the clip VI that removes the data between the cursors."
        n84 = Unbundle By Name(w231) -> ("Remove Ref"=w217:refnum<vi>, "Set Cursors Ref"=w218:refnum<vi>, "Edit File Ref"=w235:refnum<vi>, "Save Ref"=w234:refnum<vi>, "Audio"=w232:dynamicdata, "Pressure"=w224:dynamicdata, "Flow"=w223:dynamicdata)
        n85 = Build Array(w217, w218) -> (w220:refnum<vi>[])
        n86 = Build Array(w235, w234) -> (w237:refnum<vi>[])
        n87 = call "Set Enable State on Multiple Controls.vi"("Enable?"=FALSE, "Controls"=w220) -> ()  [unwired: 10 in]
        n88 = call "Set Enable State on Multiple Controls.vi"("Enable?"=TRUE, "Controls"=w237) -> ()  [unwired: 10 in]
        n89 = local read "Right"() -> (w225:dbl)
        n90 = local read "Left"() -> (w226:dbl)
        n91 = call "Remove Between Cursors.vi"("Left"=w226, "Right"=w225, "error in (no error)"=w227, "Flow"=w223, "Pressure"=w224, "Audio"=w232) -> ("error out"=w228:errorcluster, "Flow Clipped"=w221:dynamicdata, "Pressure Clipped"=w222:dynamicdata, "Audio Clipped"=w229:dynamicdata)  [unwired: 2 in]
        n92 = Bundle By Name(cluster=w231, "Audio"=w229, "Pressure"=w222, "Flow"=w221) -> (w230:T1)
        n93 = call-poly "Enqueue Message.vi"("error in (no error)"=w228, "Message Data"="Removing the selected data" ("\"Do Something Else\" button pressed"), "Message"="Update Display", "Message Queue"=w238) -> ("error out"=w239:errorcluster)  [unwired: 6 in, 1 out]
      }
      frame "Update Display" {
        # "Updates the message display."
        n94 = Unbundle By Name(w247) -> ("File Name Display"=w246:string, "Audio"=w245:dynamicdata, "Pressure"=w244:dynamicdata, "Flow"=w243:dynamicdata)
        n95 = Variant To Data(error in=w252, type="", Variant=w251) -> (data=→"Message":string, error out=w249:errorcluster)
        n96 = local write "Audio"(w245) -> ()
        n97 = local write "Flow"(w243) -> ()
        n98 = local write "File Name Display"(w246) -> ()
        n99 = local write "Pressure"(w244) -> ()
        n100 = Merge Errors(w249) -> (w253:errorcluster)
      }
      frame "Error" {
        # "Error - Check the error message data and respond accordingly. This message is sent by the \"Error Handler\" VIs at the end of each loop in this application."
        n101 = Variant To Data(error in=w265, type=errorcluster {"status"=FALSE, "code"=0, "source"=""} ("error constant"), Variant=w263) -> (data=w261:errorcluster, error out=w260:errorcluster)
        n102 = call-poly "Enqueue Message.vi"("Priority Message? (F)"=TRUE, "Message"="Exit", "Message Queue"=w257) -> ("error out"=w259:errorcluster)  [unwired: 7 in, 1 out]
        n103 = call <vilib>:"Simple Error Handler.vi"("error in (no error)"=w261) -> ()  [unwired: 4 in, 5 out]
        n104 = Merge Errors(w259, w260) -> (w258:errorcluster)
      }
      frame "Confirm Quit" {
        # "Confirm Quit - Message that can confirm whether or not the user wants to exit the application."
        n105 = call-poly "Enqueue Message.vi"("Priority Message? (F)"=TRUE, "error in (no error)"=w273, "Message"="Exit", "Message Queue"=w269) -> ("error out"=w270:errorcluster)  [unwired: 6 in, 1 out]
        n106 = Merge Errors(w270) -> (w271:errorcluster)
      }
      frame "---Copy This Frame---" {
        # "Duplicate this frame when creating new messages.  Change this comment in the duplicated frame to describe this message."
        n107 = Merge Errors(w277) -> (w275:errorcluster)
      }
      frame "Hush" {
        n108 = Merge Errors(w281) -> (w279:errorcluster)
      }
      frame "Exit" {
        # "Exit - Exit the application."
        n109 = Release Queue(queue=w291, error in (no error)=w286) -> (error out=w288:errorcluster)  [unwired: 1 in, 2 out]
        n110 = call "Fire User Event - Stop.vi"("User Event - Stop"=w285) -> ("error out"=w284:errorcluster)  [unwired: 10 in]
        n111 = local write "Stop Everything?"(TRUE ("Stop Everything?")) -> ()
        n112 = Merge Errors(w284, w288) -> (w287:errorcluster)
      }
      frame Default {
        # "'Default' case only runs if there is a message that isn't defined in any of the other cases.  Output a programming error."
        n113 = xnode "Error Ring"("parameter 0"=w293) -> ("error out"=w294:errorcluster)
      }
    }
    n114 = call "Error Handler - Message Handling Loop.vi"("error in (no error)"=w21, "Message Queue"=w23) -> ("dup error in"=w22:errorcluster)  [unwired: 8 in, 1 out]
  }
  n115 = while {
    tunnel: w6 -> [w309]
    tunnel: [w307] -> w10
    stop <- "Stop Everything?" stop-if-true
    # "Cursor Loop - Controls cursor position. Pressure and Flow positions depend on the Audio positions."
    n116 = property on="Audio" class="WFGraph (strict)"(error in=w309) -> (error out=w308:errorcluster, "CrsrList"=w310:T2)  [unwired: 1 in, 1 out]
    n117 = Array To Cluster(array=w310) -> (cluster=w305:T6)
    n118 = Unbundle By Name(w305) -> ("CrsrList[0].Position.X"=w312:dbl, "CrsrList[1].Position.X"=w306:dbl)
    "Left" <- w312
    "Right" <- w306
    n119 = Bundle By Name(cluster=w305, "CrsrList[0].Position.X"=w312, "CrsrList[1].Position.X"=w306) -> (w304:T6)
    n120 = Cluster To Array(cluster=w304) -> (array=w303:T5)
    n121 = property on="Pressure" class="WFGraph (strict)"(error in=w308, "CrsrList"=w303) -> (error out=w311:errorcluster)  [unwired: 1 in, 1 out]
    n122 = property on="Flow" class="WFGraph (strict)"(error in=w311, "CrsrList"=w303) -> (error out=w307:errorcluster)  [unwired: 1 in, 1 out]
  }
  n123 = while {
    tunnel: w16 -> [w320]
    shift-right: [w318] -> w12
    shift-left: w15 -> [w319]
    tunnel: [w314] -> w11
    stop <- w316 stop-if-true
    # "Event Handling Loop"
    n124 = event shown="[9] Key Down" {
      selector: w319 -> [_ _ _ _ _ _ _ _ _ _]
      dyn-events: [_ _ _ _ _ _ _ _ _ _] -> w318
      timeout: _ -> [_ _ _ _ _ _ _ _ _ _]
      tunnel: [_ _ _ _ _ _ _ _ TRUE ("Discard?") _] -> w316
      tunnel: w320 -> [w324 w328 w331 w335 w339 w345 w347 w352 w355 w358]
      tunnel: [w321 w325 w330 w334 w337 w344 _ w351 _ w356] -> w317
      tunnel: [w323 w327 w329 w333 w338 w343 w347 w350 w355 w357] -> w315
      event "Open": Value Change {
        n125 = event-data() -> ()  [unwired: 1 in, 1 out]
        n126 = call-poly "Enqueue Message.vi"("Message"="Open File", "Message Queue"=w324) -> ("error out"=w321:errorcluster, "dup Message Queue"=w323:refnum<queue>)  [unwired: 8 in]
      }
      event "Save": Value Change {
        n127 = event-data() -> ()  [unwired: 1 in, 1 out]
        n128 = call-poly "Enqueue Message.vi"("Message"="Save File", "Message Queue"=w328) -> ("error out"=w325:errorcluster, "dup Message Queue"=w327:refnum<queue>)  [unwired: 8 in]
      }
      event "Edit File": Value Change {
        n129 = event-data() -> ()  [unwired: 1 in, 1 out]
        n130 = call-poly "Enqueue Message.vi"("Message"="Edit File", "Message Queue"=w331) -> ("error out"=w330:errorcluster, "dup Message Queue"=w329:refnum<queue>)  [unwired: 8 in]
      }
      event "Set Cursors": Value Change {
        n131 = event-data() -> ()  [unwired: 1 in, 1 out]
        n132 = call-poly "Enqueue Message.vi"("Message"="Set Cursors", "Message Queue"=w335) -> ("error out"=w334:errorcluster, "dup Message Queue"=w333:refnum<queue>)  [unwired: 8 in]
      }
      event "Remove": Value Change {
        n133 = event-data() -> ()  [unwired: 1 in, 1 out]
        n134 = call-poly "Enqueue Message.vi"("Message"="Remove", "Message Queue"=w339) -> ("error out"=w337:errorcluster, "dup Message Queue"=w338:refnum<queue>)  [unwired: 8 in]
      }
      event Panel Close? {
        n135 = event-data() -> ()  [unwired: 1 in, 1 out]
        n136 = call-poly "Enqueue Message.vi"("Priority Message? (F)"=TRUE, "Message"="Confirm Quit", "Message Queue"=w345) -> ("error out"=w344:errorcluster, "dup Message Queue"=w343:refnum<queue>)  [unwired: 7 in]
        n137 = event-data("Discard?"=TRUE) -> ()  [unwired: 1 in, 1 out]
      }
      event Application Instance Close {
        n138 = event-data() -> ()  [unwired: 1 in, 1 out]
      }
      event "Exit": Value Change {
        n139 = event-data() -> ()  [unwired: 1 in, 1 out]
        n140 = call-poly "Enqueue Message.vi"("Priority Message? (F)"=TRUE, "Message"="Exit", "Message Queue"=w352) -> ("error out"=w351:errorcluster, "dup Message Queue"=w350:refnum<queue>)  [unwired: 7 in]
      }
      event User Event {
        # "The Message Handling Loop processed an \"Exit\" message, which fired this event to stop the Event Handling Loop."
        n141 = event-data() -> ()  [unwired: 1 in, 1 out]
        n142 = local write "Message"("Goodbye" ("VI Stopped")) -> ()
      }
      event Key Down {
        n143 = event-data() -> ("VKey"=w359:T7)  [unwired: 1 in, 2 out]
        n144 = case shown="\"Enter\", Default" w359 {
          tunnel: w358 -> [w360 w363]
          tunnel: [w360 w364] -> w357
          tunnel: [_ w361] -> w356
          frame "Enter", Default {
          }
          frame "Home" {
            n145 = call-poly "Enqueue Message.vi"("Message"="Hush", "Message Queue"=w363) -> ("error out"=w361:errorcluster, "dup Message Queue"=w364:refnum<queue>)  [unwired: 8 in]
          }
        }
      }
    }
    n146 = call "Error Handler - Event Handling Loop.vi"("error in (no error)"=w317, "Message Queue"=w315) -> ("dup error in"=w314:errorcluster)  [unwired: 8 in, 1 out]
  }
  n147 = Unregister For Events(event registration refnum=w12, error in=w11) -> (error out=w13:errorcluster)
  n148 = Merge Errors(w13, w17, w10) -> (w7:errorcluster)
  n149 = call "Destroy User Event - Stop.vi"("error in (no error)"=w7, "User Event - Stop"=w14) -> ("error out"=→"error out":errorcluster)  [unwired: 9 in]
